vi "Outputs.vi"(8 "error in (no error)":errorcluster, 11 "Sonicator Module State Cluster":T1={"State"=enum."Idle", "Start Time"=timestamp(0 s since 1904-01-01), "Current Time"=timestamp(0 s since 1904-01-01), "Sonicator Module Config"={"GUID"="", "Drop Coords"={"Horizontal"=0, "Vertical"=0}, "Process Name"="", "Queue Name"="", "Settings"={"Cycle Period"=500.0, "Sonicator Type"="", "SS P100 Settings"={"VISA resource name"="", "Simulated?"=FALSE}, "Setpoint (µm)"=0.0, "Cutoff (W)"=0.0}, "Load Count"=0}, "Output Error"=FALSE, "Log Started"=FALSE, "First Iteration"=FALSE, "Data"={"Sonicator Amp Value"=0.0, "Sonicator Power Value"=0.0}, "Sonicator On?"=enum."Off"}) -> (0 "error out":errorcluster, 3 "Sonicator Module State Cluster":T1={"State"=enum."Idle", "Start Time"=timestamp(0 s since 1904-01-01), "Current Time"=timestamp(0 s since 1904-01-01), "Sonicator Module Config"={"GUID"="", "Drop Coords"={"Horizontal"=0, "Vertical"=0}, "Process Name"="", "Queue Name"="", "Settings"={"Cycle Period"=500.0, "Sonicator Type"="", "SS P100 Settings"={"VISA resource name"="", "Simulated?"=FALSE}, "Setpoint (µm)"=0.0, "Cutoff (W)"=0.0}, "Load Count"=0}, "Output Error"=FALSE, "Log Started"=FALSE, "First Iteration"=FALSE, "Data"={"Sonicator Amp Value"=0.0, "Sonicator Power Value"=0.0}, "Sonicator On?"=enum."Off"})   [LabVIEW 2018, in "Sonicator Module.lvlib" / "Sonicator Module Engine.lvlib"]
uses:
  Sonicator Module Engine.lvlib
  Feed Module/Controls/Sonicator Module State Cluster.ctl
  Pump Module Folder/Measure Instrument/State Enum.ctl
  Feed Module/Controls/Sonicator Module Config Cluster.ctl
  <vilib>/Utility/miscctls.llb/LVPoint32TypeDef.ctl
  Feed Module/Controls/Sonicator Module Settings Cluster.ctl
  Sonic Systems P100/Sonic Systems P100 Settings.ctl
  Tag VIs/Tag FGV Operation Enum.ctl
  Shared Variables/Dynamic Shared Variables.lvlib
  Sonic Systems P100/Sonic Systems P100.lvlib
  Pump Module Folder/Measure Instrument/Pump Module Engine.lvlib
  Sonicator Module.lvlib
panel:
  # "Sonicator Settings"
  # "Sonicator Settings"
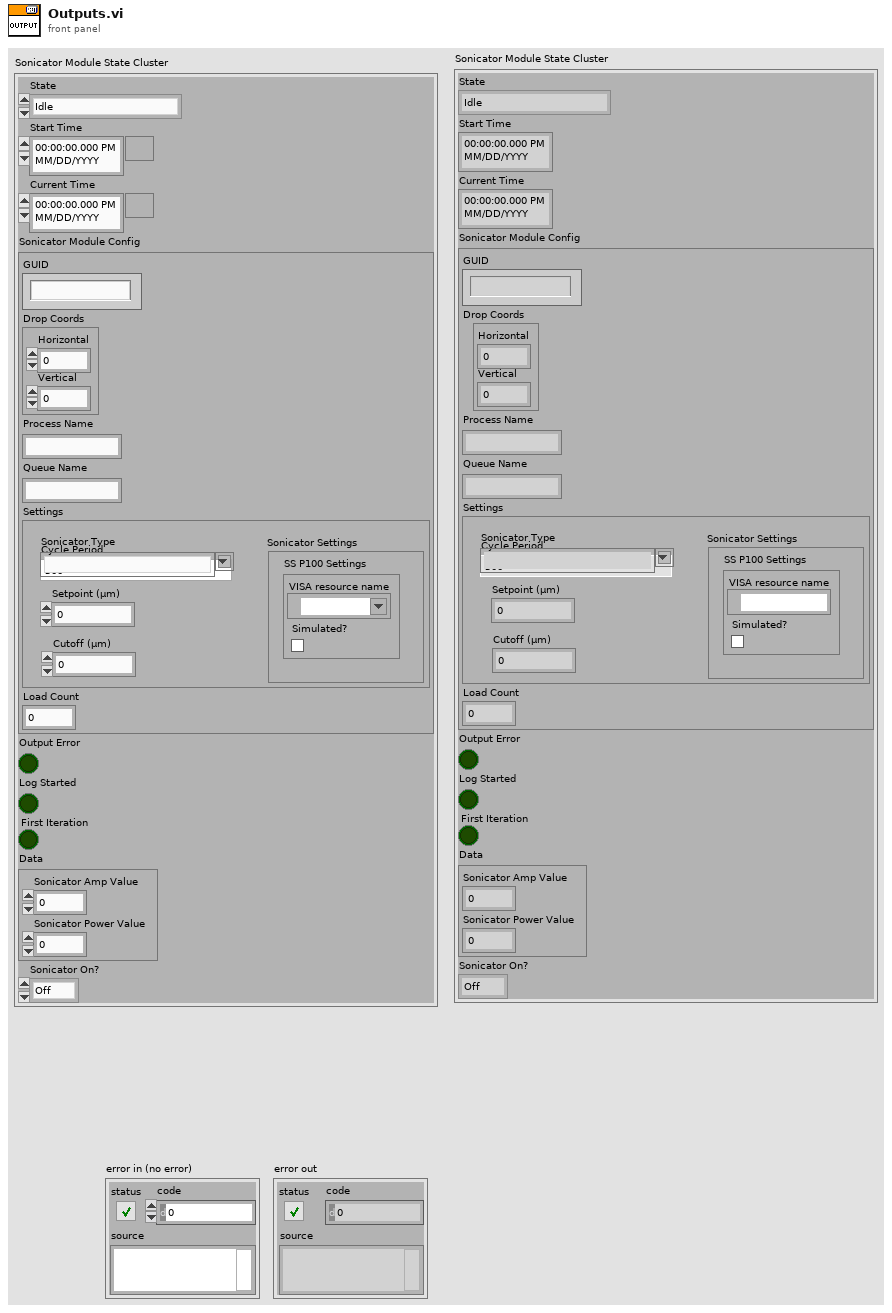
[diagram p1: front panel]
types:
  T1 = typedef "Sonicator Module.lvlib/Sonicator Module State Cluster.ctl" = cluster{"State":T2, "Start Time":timestamp, "Current Time":timestamp, "Sonicator Module Config":T3, "Output Error":bool, "Log Started":bool, "First Iteration":bool, "Data":cluster{"Sonicator Amp Value":dbl, "Sonicator Power Value":dbl}, "Sonicator On?":enum16{"Off", "On", "Not Initialized", "Over Cutoff"}}
  T2 = typedef "Pump Module.lvlib/Pump Module Engine.lvlib/State Enum.ctl" = enum16{"Measuring", "Idle", "Paused"}
  T3 = typedef "Sonicator Module.lvlib/Sonicator Module Config Cluster.ctl" = cluster{"GUID":string, "Drop Coords":T4, "Process Name":string, "Queue Name":string, "Settings":T5, "Load Count":i32}
  T4 = typedef "LVPoint32TypeDef.ctl" = cluster{"Horizontal":i32, "Vertical":i32}
  T5 = typedef "Sonicator Module.lvlib/Sonicator Module Settings Cluster.ctl" = cluster{"Cycle Period":dbl, "Sonicator Type":string, "SS P100 Settings":T6, "Setpoint (µm)":dbl, "Cutoff (W)":dbl}
  T6 = typedef "Sonic Systems P100.lvlib/Sonic Systems P100 Settings.ctl" = cluster{"VISA resource name":refnum<visa-resource-name>, "Simulated?":bool}
  T7 = typedef "Tag FGV Operation Enum.ctl" = enum16{"Init", "Set Notification Queue", "Create Tag", "Commit", "Write Tag (Numeric)", "Write Tag (Boolean)", "Read All Tags", "Read One Tag", "Delete Tag Category", "Set Alarm Parameters (Numeric)", "Set Alarm Parameters (Boolean)", "Enable All Alarms", "Disable All Alarms", "Delete All Tags", "Read Alarms", "Ack Alarm", "Read Alarm Parameters (Numeric)", "Read Alarm Parameters (Boolean)"}
  T8 = cluster{"Amplitude Tag":string, "Power Tag":string, "Output Device Tag":string}
  T9 = enum16{"Off", "On", "Not Initialized", "Over Cutoff"}
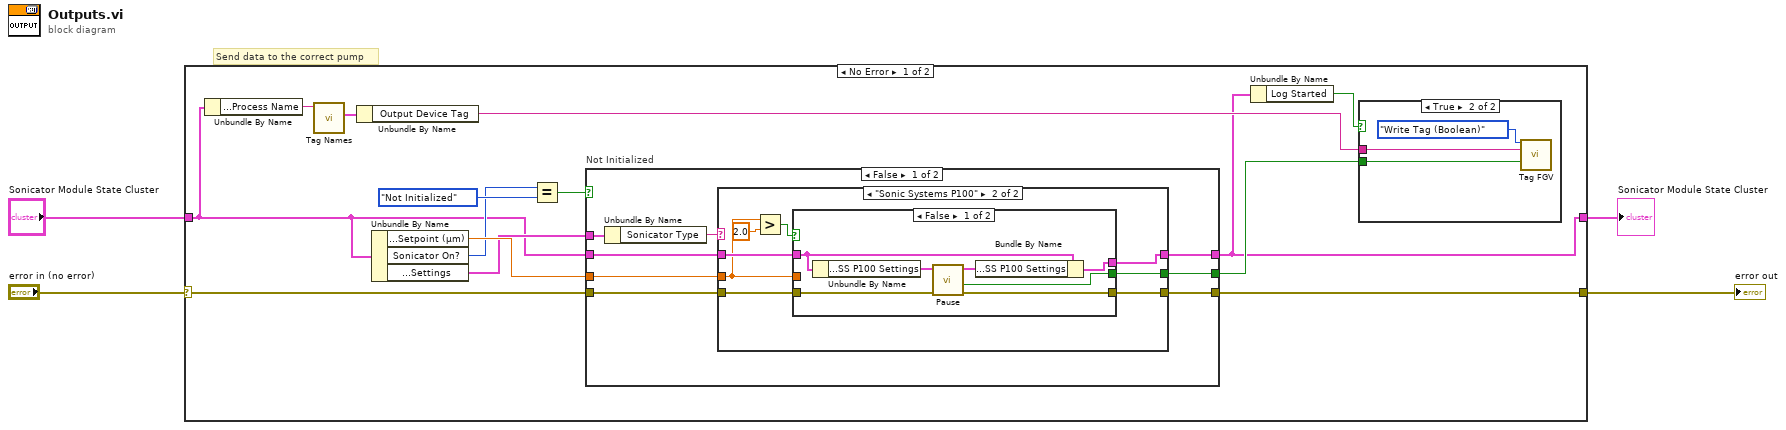
[diagram p0: block diagram]
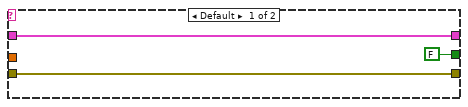
[diagram p3: hidden frame]
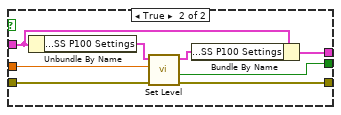
[diagram p4: hidden frame]
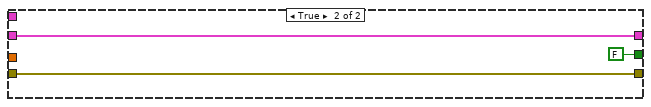
[diagram p5: hidden frame]
diagram:
  # "Send data to the correct pump"
  n1 = case shown="No Error" "error in (no error)" {
    selector: "error in (no error)" -> [w18 w60]
    tunnel: [w17 w60] -> w3
    tunnel: "Sonicator Module State Cluster" -> [w5 w59]
    tunnel: [w11 w59] -> w1
    frame No Error {
      n2 = Unbundle By Name(w5) -> ("Sonicator Module Config.Process Name"=w7:string)
      n3 = call "Tag Names.vi"("Process Name"=w7) -> ("SC Tags"=w8:T8)  [unwired: 8 in, 2 out]
      n4 = Unbundle By Name(w8) -> ("Output Device Tag"=w16:string)
      n5 = Unbundle By Name(w5) -> ("Sonicator Module Config.Settings.Setpoint (µm)"=w12:dbl, "Sonicator On?"=w9:T9, "Sonicator Module Config.Settings"=w6:T5)
      n6 = Equal?(x=w9, y=enum16{"Off", "On", "Not Initialized"}."Not Initialized" ("x")) -> (x = y?=w14:bool)
      n7 = case "Not Initialized" shown="False" w14 {
        tunnel: w18 -> [w26 w57]
        tunnel: [w25 w57] -> w17
        tunnel: [w22 FALSE ("Connection Error")] -> w15
        tunnel: w12 -> [w24 _]
        tunnel: [w27 w56] -> w11
        tunnel: w6 -> [w29 _]
        tunnel: w5 -> [w23 w56]
        frame False {
          n8 = Unbundle By Name(w29) -> ("Sonicator Type"=w28:string)
          n9 = case shown="\"Sonic Systems P100\"" w28 {
            tunnel: [w30 w38] -> w27
            tunnel: w26 -> [w32 w40]
            tunnel: [w32 w37] -> w25
            tunnel: w24 -> [_ w35]
            tunnel: w23 -> [w30 w39]
            tunnel: [FALSE ("Connection Error") w36] -> w22
            frame Default {
            }
            frame "Sonic Systems P100" {
              n10 = Greater?(x=w35, y=2.0) -> (0:w33:bool)
              n11 = case shown="False" w33 {
                tunnel: w40 -> [w47 w55]
                tunnel: w35 -> [_ w54]
                tunnel: w39 -> [w42 w52]
                tunnel: [w41 w50] -> w38
                tunnel: [w46 w49] -> w37
                tunnel: [w45 w48] -> w36
                frame False {
                  n12 = Unbundle By Name(w42) -> ("Sonicator Module Config.Settings.SS P100 Settings"=w43:T6)
                  n13 = call "Pause.vi"("error in (no error)"=w47, "SS P100 Settings In"=w43) -> ("error out"=w46:errorcluster, "Connection Error"=w45:bool, "SS P100 Settings Out"=w44:T6)  [unwired: 7 in]
                  n14 = Bundle By Name(cluster=w42, "Sonicator Module Config.Settings.SS P100 Settings"=w44) -> (w41:T1)
                }
                frame True {
                  n15 = Unbundle By Name(w52) -> ("Sonicator Module Config.Settings.SS P100 Settings"=w53:T6)
                  n16 = call "Set Level.vi"("error in (no error)"=w55, "Setpoint"=w54, "SS P100 Settings In"=w53) -> ("error out"=w49:errorcluster, "Connection Error"=w48:bool, "SS P100 Settings Out"=w51:T6)  [unwired: 6 in]
                  n17 = Bundle By Name(cluster=w52, "Sonicator Module Config.Settings.SS P100 Settings"=w51) -> (w50:T1)
                }
              }
            }
          }
        }
        frame True {
        }
      }
      n18 = Unbundle By Name(w11) -> ("Log Started"=w13:bool)
      n19 = case shown="True" w13 {
        tunnel: w16 -> [_ w21]
        tunnel: w15 -> [_ w20]
        frame False {
        }
        frame True {
          n20 = call "Tag FGV.vi"("Operation"=Tag_FGV_Operation_Enum."Write Tag (Boolean)", "Tag Name"=w21, "Data"=w20) -> ()  [unwired: 5 in, 8 out]
        }
      }
    }
    frame Error {
    }
  }
  "error out" <- w3
  "Sonicator Module State Cluster" <- w1
